vi "Parse DB RX Labels.vi"(8 "error in":errorcluster, 11 "config handle":u32) -> (0 "error out":errorcluster, 2 "Labels":T1[](array[typedef]) {"scheduleBuildUnit" items=["Millisecond", "Microsecond"]})   [LabVIEW 2016]
uses:
  Controls/AIT_Label.ctl
  Controls/AIT_Word.ctl
  Controls/ARINCParam.ctl
  Shared/Controls and Global/TransferType.ctl
  Ballard Arinc-429 System Explorer.lvlib
  <userlib>/ARINC-429/Owl429.lvlib
  Shared/Ballard Arinc-429 Shared.lvlib
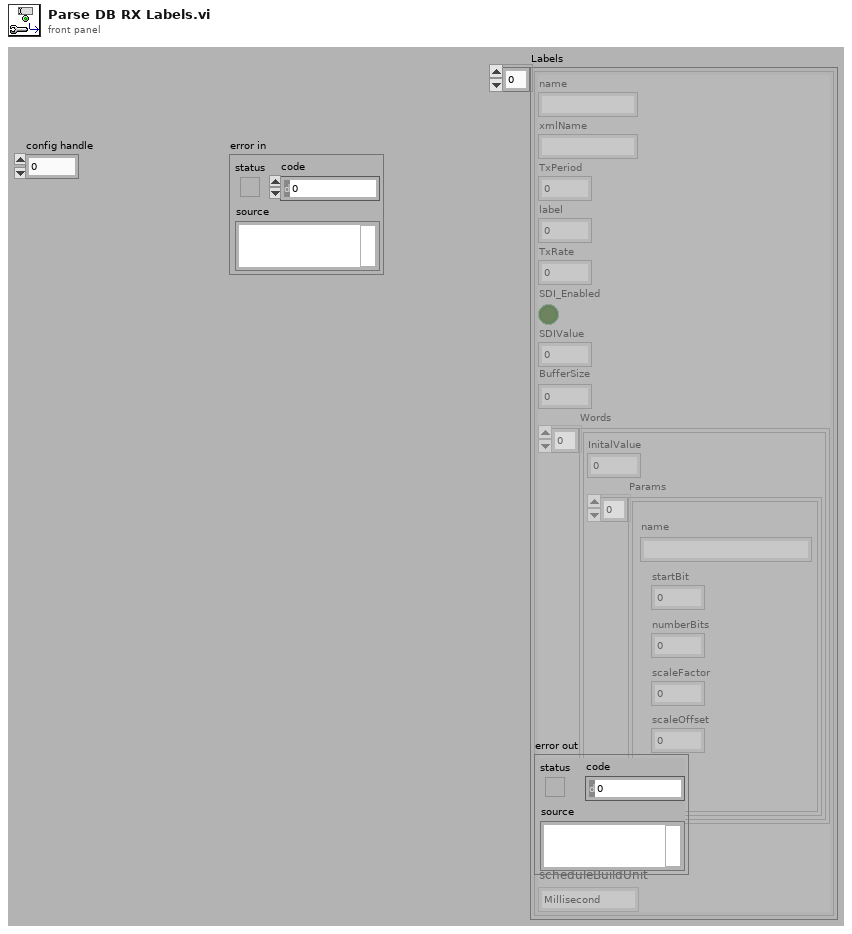
[diagram p1: front panel]
types:
  T1 = typedef "Ballard Arinc-429 System Explorer.lvlib/AIT_Label.ctl" = cluster{"name":string, "xmlName":string, "TxPeriod":u32, "label":u32, "TxRate":dbl, "SDI_Enabled":bool, "SDIValue":u8, "BufferSize":u32, "Words":T2[], "TransferType":T4, "scheduleBuildUnit":i32}
  T2 = typedef "Ballard Arinc-429 System Explorer.lvlib/AIT_Word.ctl" = cluster{"InitalValue":u32, "Params":T3[]}
  T3 = typedef "Ballard Arinc-429 System Explorer.lvlib/ARINCParam.ctl" = cluster{"name":string, "startBit":i32, "numberBits":i32, "scaleFactor":dbl, "scaleOffset":dbl, "signed":bool}
  T4 = typedef "Ballard Arinc-429 Shared.lvlib/TransferType.ctl" = enum16{"ScheduledLabel", "Acyclic", "Block", "Strobe"}
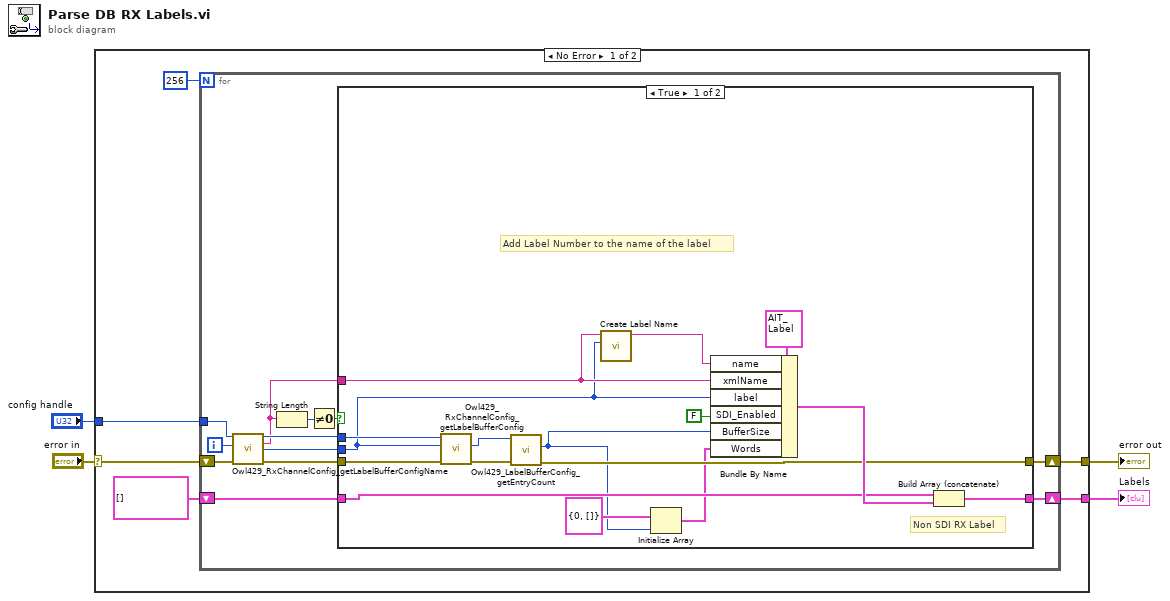
[diagram p0: block diagram]
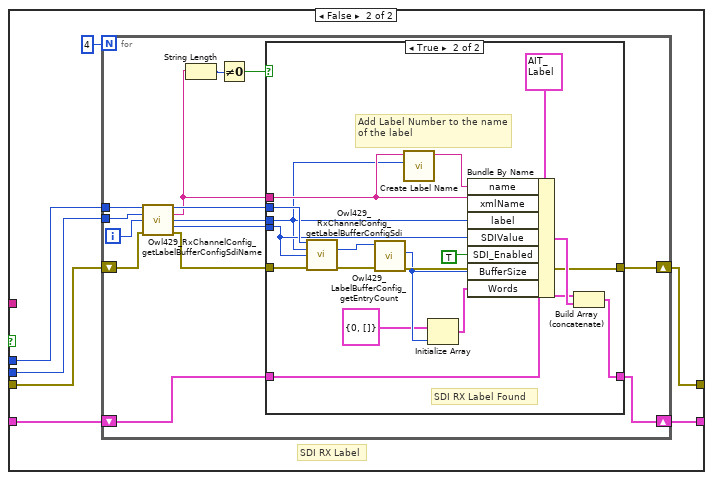
[diagram p2: hidden frame]
diagram:
  n1 = case shown="No Error" "error in" {
    selector: "error in" -> [w6 w79]
    tunnel: [w10 _] -> w1
    tunnel: [w9 w79] -> w2
    tunnel: "config handle" -> [w8 _]
    frame No Error {
      n2 = for {
        N: 256 -> [_]
        shift-right: [w20] -> w9
        shift-left: w6 -> [w16]
        tunnel: w8 -> [w18]
        shift-right: [w22] -> w10
        shift-left: T1[] [] -> [w21]
        i -> [w17]
        n3 = call <userlib>:"Owl429_RxChannelConfig_getLabelBufferConfigName.vi"("rx channel config handle"=w18, "label"=w17, "error in (no error)"=w16) -> ("rx channel config handle"=w14:u64, "label buffer config name"=w12:string, "label"=w13:u8, "error out"=w15:errorcluster)  [unwired: 9 in]
        n4 = String Length(string=w12) -> (length=w11:i32)
        n5 = Not Equal To 0?(x=w11) -> (x != 0?=w19:bool)
        n6 = case shown="True" w19 {
          tunnel: [w38 w40] -> w22
          tunnel: [w28 w39] -> w20
          tunnel: w15 -> [w29 w41]
          tunnel: w14 -> [w27 w43]
          tunnel: w13 -> [w26 w42]
          tunnel: w21 -> [w34 w45]
          tunnel: w12 -> [w32 _]
          frame True {
            # "Add Label Number to the name of the label"
            # "Non SDI RX Label"
            n7 = call <userlib>:"Owl429_RxChannelConfig_getLabelBufferConfig.vi"("error in (no error)"=w29, "label"=w26, "rx channel config handle"=w27) -> ("error out"=w30:errorcluster, "label buffer config handle"=w31:u64)  [unwired: 5 in, 2 out]
            n8 = call <userlib>:"Owl429_LabelBufferConfig_getEntryCount.vi"("error in (no error)"=w30, "label buffer config handle"=w31) -> ("error out"=w28:errorcluster, "entry count"=w23:u32)  [unwired: 7 in, 1 out]
            n9 = call "Create Label Name.vi"("label number"=w26, "label XML name"=w32) -> ("label name"=w33:string)  [unwired: 9 in]
            n10 = Initialize Array(T2 {"InitalValue"=0, "Params"=[]} ("Word"), w23) -> (w24:T2[])
            n11 = Bundle By Name(cluster=T1 {"name"="", "xmlName"="", "TxPeriod"=0, "label"=0, "TxRate"=0.0, "SDI_Enabled"=FALSE, "SDIValue"=0, "BufferSize"=0, "Words"=[], "TransferType"=enum."ScheduledLabel", "scheduleBuildUnit"=0} ("Label"), "name"=w33, "xmlName"=w32, "label"=w26, "SDI_Enabled"=FALSE, "BufferSize"=w23, "Words"=w24) -> (w36:T1)
            n12 = Build Array (concatenate)(w34, w36) -> (w38:T1[])
          }
          frame False {
            # "SDI RX Label"
            n13 = for {
              N: 4 -> [_]
              tunnel: w43 -> [w50]
              tunnel: w42 -> [w49]
              shift-right: [w59] -> w39
              shift-left: w41 -> [w48]
              shift-right: [w57] -> w40
              shift-left: w45 -> [w58]
              i -> [w46]
              n14 = call <userlib>:"Owl429_RxChannelConfig_getLabelBufferConfigSdiName.vi"("rx channel config handle"=w50, "label"=w49, "sdi"=w46, "error in (no error)"=w48) -> ("rx channel config handle"=w56:u64, "label buffer config name"=w54:string, "label"=w51:u8, "sdi"=w52:u8, "error out"=w47:errorcluster)  [unwired: 7 in]
              n15 = String Length(string=w54) -> (length=w53:i32)
              n16 = Not Equal To 0?(x=w53) -> (x != 0?=w55:bool)
              n17 = case shown="True" w55 {
                tunnel: w47 -> [w60 w72]
                tunnel: w56 -> [_ w70]
                tunnel: [w60 w71] -> w59
                tunnel: w58 -> [w61 w76]
                tunnel: [w61 w75] -> w57
                tunnel: w54 -> [_ w69]
                tunnel: w52 -> [_ w68]
                tunnel: w51 -> [_ w67]
                frame False {
                }
                frame True {
                  # "Add Label Number to the name of the label"
                  # "SDI RX Label Found"
                  n18 = call <userlib>:"Owl429_RxChannelConfig_getLabelBufferConfigSdi.vi"("rx channel config handle"=w70, "label"=w67, "sdi"=w68, "error in (no error)"=w72) -> ("label buffer config handle"=w66:u64, "error out"=w65:errorcluster)  [unwired: 7 in, 3 out]
                  n19 = call <userlib>:"Owl429_LabelBufferConfig_getEntryCount.vi"("error in (no error)"=w65, "label buffer config handle"=w66) -> ("error out"=w71:errorcluster, "entry count"=w64:u32)  [unwired: 7 in, 1 out]
                  n20 = call "Create Label Name.vi"("label number"=w67, "label XML name"=w69) -> ("label name"=w73:string)  [unwired: 9 in]
                  n21 = Initialize Array(T2 {"InitalValue"=0, "Params"=[]} ("Word"), w64) -> (w62:T2[])
                  n22 = Bundle By Name(cluster=T1 {"name"="", "xmlName"="", "TxPeriod"=0, "label"=0, "TxRate"=0.0, "SDI_Enabled"=FALSE, "SDIValue"=0, "BufferSize"=0, "Words"=[], "TransferType"=enum."ScheduledLabel", "scheduleBuildUnit"=0} ("Label"), "name"=w73, "xmlName"=w69, "label"=w67, "SDIValue"=w68, "SDI_Enabled"=TRUE, "BufferSize"=w64, "Words"=w62) -> (w78:T1)
                  n23 = Build Array (concatenate)(w76, w78) -> (w75:T1[])
                }
              }
            }
          }
        }
      }
    }
    frame Error {
    }
  }
  "Labels" <- w1
  "error out" <- w2
